vi "calc com end of volume2.vi"(10 "end of volume":bool, 11 "running sums in":T1) -> (0 "ready for input":bool, 1 "output valid":bool, 2 "center of mass":cluster{"x avg":i16, "y avg":i16, "z avg":i16}, 3 "running sums out":T1)   [LabVIEW 2010]
uses:
  <vilib>/rvi/FXPMathLib/FxpReciprocal/XNode/nifxpmath_Reciprocal.xnode
  <vilib>/rvi/FXPMathLib/FxpDiv/XNode/nifxpmath_Div.xnode
  <vilib>/rvi/FXPMathLib/FxpDiv/subVIs/nifxpmath_Div_SimConfig.ctl
  <vilib>/rvi/FXPMathLib/FxpMul/XNode/nifxpmath_Multiplier.xnode
  <vilib>/rvi/FXPMathLib/FxpMul/subVIs/nifxpmath_Mul_SimConfig.ctl
  <vilib>/fxp/LVFixedPointQuantizationPolicyTypeDef.ctl
  <vilib>/fxp/LVFixedPointOverflowPolicyTypeDef.ctl
  <vilib>/rvi/FXPMathLib/FxpDiv/simVIs/DllFxpDivTemp_sub.vi
  <vilib>/rvi/FXPMathLib/FxpMul/simVIs/DllFxpMulTemp_sub.vi
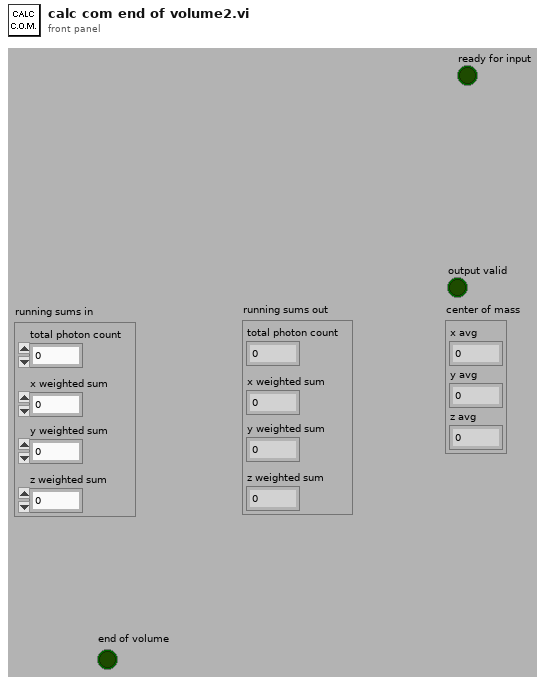
[diagram p1: front panel]
types:
  T1 = cluster{"total photon count":u32, "x weighted sum":i32, "y weighted sum":i32, "z weighted sum":i32}
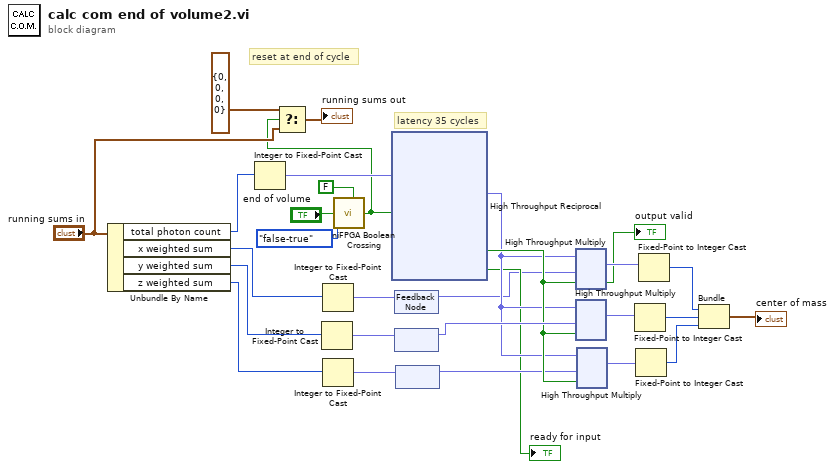
[diagram p0: block diagram]
diagram:
  # "reset at end of cycle"
  # "latency 35 cycles"
  n1 = Unbundle By Name("running sums in") -> ("total photon count"=w16:u32, "x weighted sum"=w6:i32, "y weighted sum"=w15:i32, "z weighted sum"=w2:i32)
  n2 = Integer to Fixed-Point Cast(integer=w16) -> (fixed-point=w29:fxp<+,32,32>)  [unwired: 1 in]
  n3 = Integer to Fixed-Point Cast(integer=w15) -> (fixed-point=w25:fxp<+/-,32,32>)  [unwired: 1 in]
  n4 = Integer to Fixed-Point Cast(integer=w6) -> (fixed-point=w5:fxp<+/-,32,32>)  [unwired: 1 in]
  n5 = Integer to Fixed-Point Cast(integer=w2) -> (fixed-point=w24:fxp<+/-,32,32>)  [unwired: 1 in]
  n6 = call <vilib>:"niFPGA Boolean Crossing.vi"("input"="end of volume", "direction"=enum8{"either", "false-true", "true-false"}."false-true", "initialize"=FALSE) -> ("crossing"=w3:bool)  [unwired: 6 in]
  n7 = Select(t=T1 {"total photon count"=0, "x weighted sum"=0, "y weighted sum"=0, "z weighted sum"=0} ("running sums out"), s=w3, f="running sums in") -> (s? t:f=→"running sums out":T1)
  n8 = xnode "High Throughput Reciprocal"("x"=w29, "input valid"=w3) -> ("1/x"=w20:fxp<+,32,0>, "output valid"=w22:bool, "ready for input"=→"ready for input":bool)  [unwired: 1 in]
  n9 = feedback-in #1(w5) -> ()
  n10 = feedback #1() -> (w4:fxp<+/-,32,32>)  [unwired: 1 in]
  n11 = feedback #2() -> (w23:fxp<+/-,32,32>)  [unwired: 1 in]
  n12 = feedback-in #2(w25) -> ()
  n13 = feedback #3() -> (w21:fxp<+/-,32,32>)  [unwired: 1 in]
  n14 = feedback-in #3(w24) -> ()
  n15 = xnode "High Throughput Multiply"("x"=w20, "y"=w4, "input valid"=w22) -> ("x*y"=w19:fxp<+/-,16,16>, "output valid"=→"output valid":bool)  [unwired: 1 in, 1 out]
  n16 = xnode "High Throughput Multiply"("x"=w20, "y"=w23, "input valid"=w22) -> ("x*y"=w18:fxp<+/-,16,16>)  [unwired: 1 in, 2 out]
  n17 = xnode "High Throughput Multiply"("x"=w20, "y"=w21, "input valid"=w22) -> ("x*y"=w17:fxp<+/-,16,16>)  [unwired: 1 in, 2 out]
  n18 = Fixed-Point to Integer Cast(1:w18) -> (0:w9:i16)
  n19 = Fixed-Point to Integer Cast(1:w17) -> (0:w8:i16)
  n20 = Fixed-Point to Integer Cast(1:w19) -> (0:w10:i16)
  n21 = Bundle(w10, w9, w8) -> (→"center of mass":cluster{i16, i16, i16})  [unwired: 1 in]
